vi "MC collect shot data from tcp queue.vi"(6 "Scan.ShotDataQueuesAndEvents.tcp data event":T1, 7 "TCP subscriptions info":T2, 8 "error in (no error)":errorcluster, 9 "timeout for get all devs (ms)":u32=5000, 10 "ScanData event reg ref":refnum<event-registration>, 11 "TCPshotDataQueue":refnum<queue>) -> (0 "error out":errorcluster, 1 "timeout":bool, 2 "device times":cluster{"Device":string, "time":u32}[](array[cluster]), 3 "All data out":string[][](array[string]))   [LabVIEW 2020]
uses:
  Shared/GUI_Template/TCP subscription info cluster.ctl
  Shared/GUI_Template/GUI_master/tcp_new_data_event.ctl
  Shared/GUI_Template/GUI_master/tcp new data cluster.ctl
panel:
  out "number of events discarded":u32
  out "device times all data received":cluster{"Device":string, "time":u32}[](array[cluster])
  out "dev times timeout":cluster{"Device":string, "time":u32}[](array[cluster])
  out "time waited":u32(graph)
  out "timeout":bool
  out "time":u32 caption="time waiting"
  out "Devs no data":string[](array[string])
  out "loop time":u32
  out "Device name":string
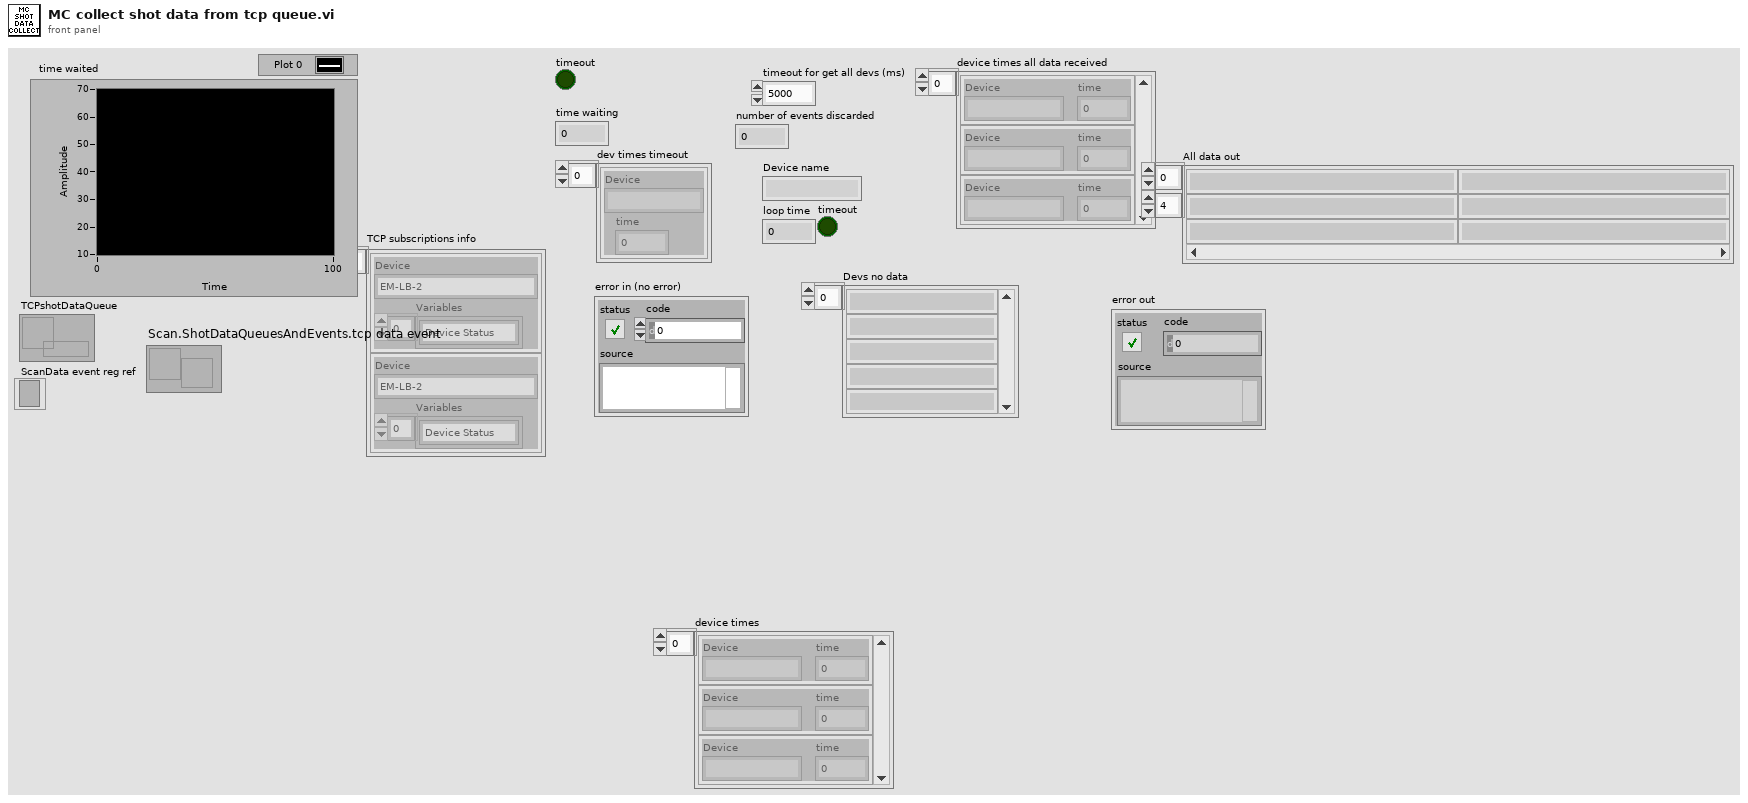
[diagram p1: front panel]
types:
  T1 = typedef "tcp_new_data_event.ctl" = refnum<user-event>
  T2 = typedef "TCP subscription info cluster.ctl" = cluster{"Device":string, "Variables":string[]}[]
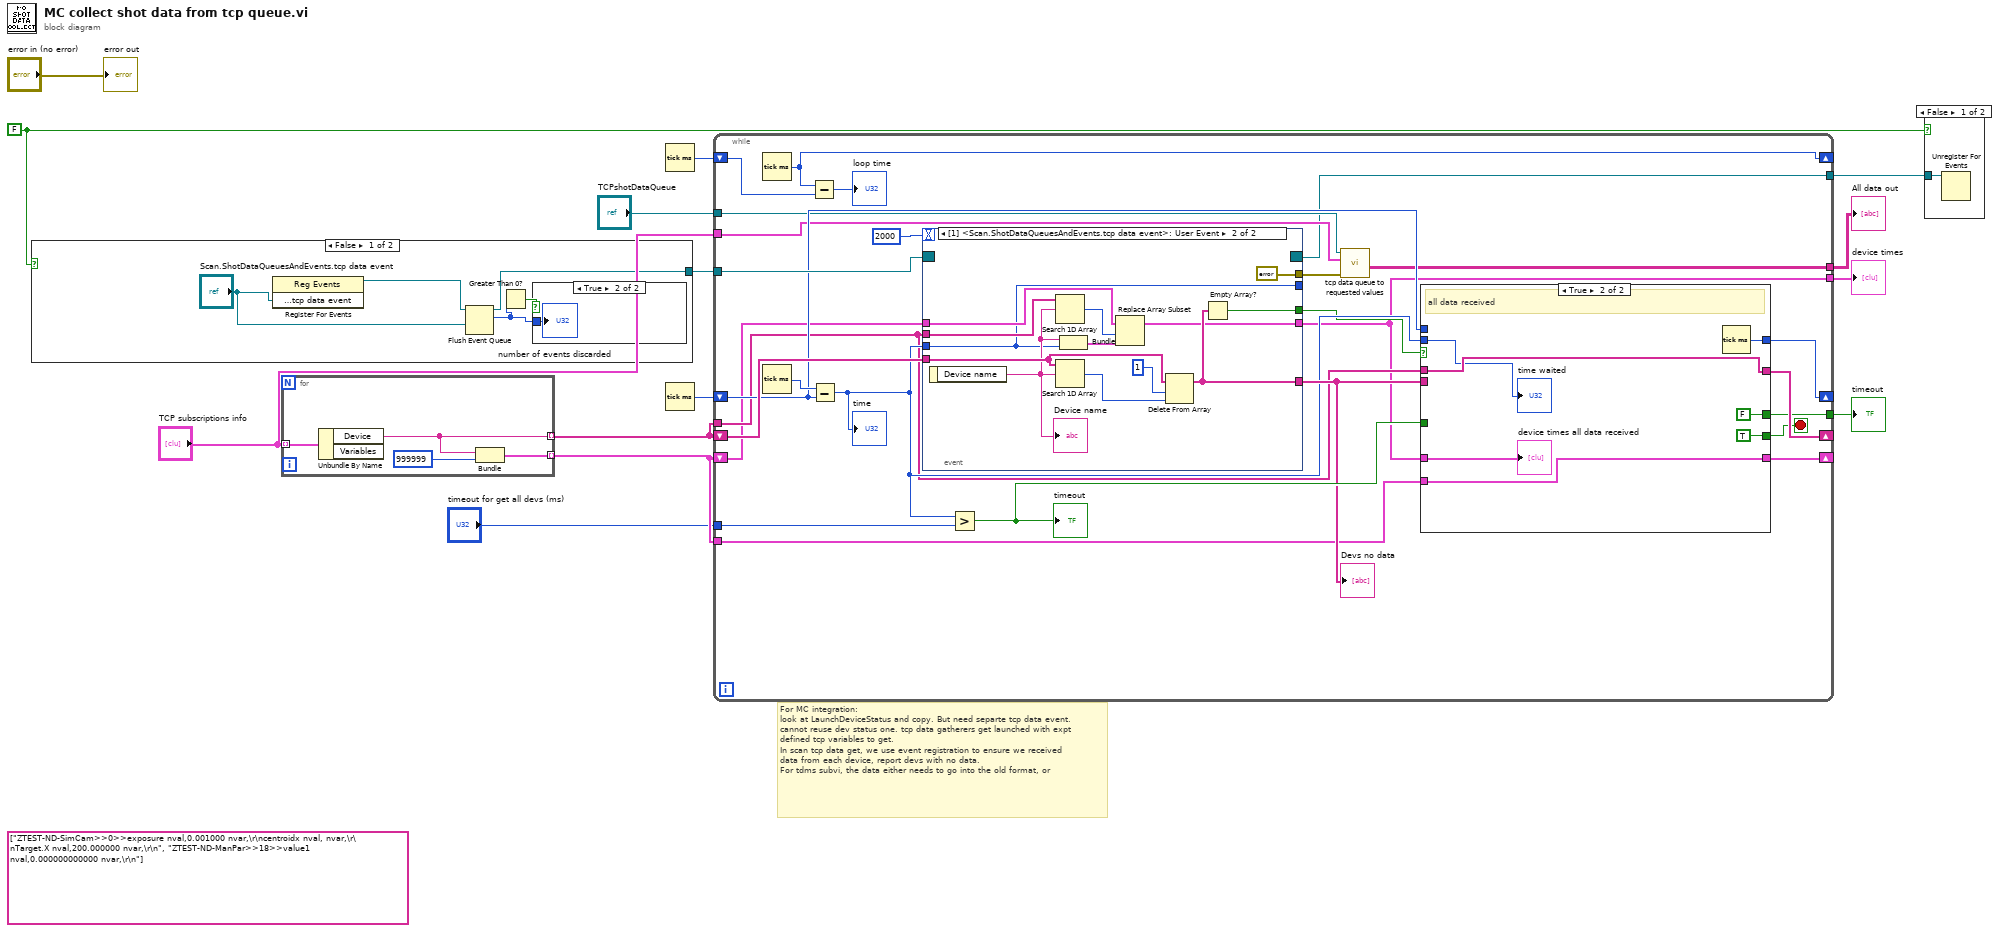
[diagram p0: block diagram]
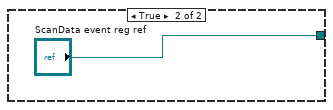
[diagram p3: hidden frame]
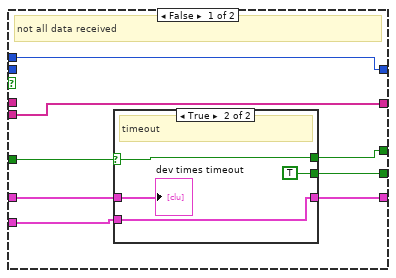
[diagram p5: hidden frame]
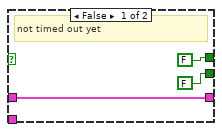
[diagram p6: hidden frame]
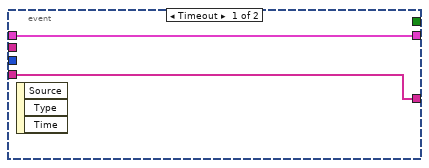
[diagram p7: hidden frame]
diagram:
  w2 = FALSE
  (unwired) string[] ["ZTEST-ND-SimCam>>0>>exposure nval,0.001000 nvar,\r\ncentroidx nval, nvar,\r\nTarget.X nval,200.000000 nvar,\r\n", "ZTEST-ND-ManPar>>18>>value1 nval,0.000000000000 nvar,\r\n"] ("Scan data in")
  # "For MC integration:\nlook at LaunchDeviceStatus and copy. But need separte tcp data event. cannot reuse dev status one. tcp data gatherers get launched with expt defined tcp variables to get.\nIn scan tcp data get, we use event registration to ensure we received data from each device, report devs with no data.\nFor tdms subvi, the data either needs to go into the old format, or"
  n1 = case shown="False" w2 {
    tunnel: [w17 "ScanData event reg ref"] -> w3
    frame False {
      n2 = register-events("Scan.ShotDataQueuesAndEvents.tcp data event") -> (reference out=w19:refnum<event-registration>)  [unwired: 2 in, 1 out]
      n3 = Flush Event Queue(0:w19, 2:"Scan.ShotDataQueuesAndEvents.tcp data event") -> (8:w17:refnum<event-registration>, 9:w16:u32)  [unwired: 4 in, 1 out]
      n4 = Greater Than 0?(x=w16) -> (x > 0?=w15:bool)
      n5 = case shown="True" w15 {
        tunnel: w16 -> [_ w20]
        frame False {
        }
        frame True {
          "number of events discarded" <- w20
        }
      }
    }
    frame True {
    }
  }
  n6 = for {
    tunnel: "TCP subscriptions info" -> [w25] mode=indexing
    tunnel: [w24] -> w12 mode=indexing
    tunnel: [w22] -> w10 mode=indexing
    n7 = Unbundle By Name(w25) -> ("Device"=w24:string)  [unwired: 1 out]
    n8 = Bundle("Device"=w24, "time"=u32 999999) -> (w22:cluster{"Device":string, "time":u32})  [unwired: 1 in]
  }
  n9 = Tick Count (ms)() -> (millisecond timer value=w14:u32)
  n10 = Tick Count (ms)() -> (millisecond timer value=w11:u32)
  n11 = while {
    tunnel: "TCPshotDataQueue" -> [w31]
    tunnel: "TCP subscriptions info" -> [w32]
    tunnel: w3 -> [w52]
    shift-right: [w50] -> _
    shift-left: w14 -> [w49]
    shift-right: [w41] -> _
    shift-left: w12 -> [w47]
    tunnel: w12 -> [w39]
    shift-right: [w45] -> _
    shift-left: w11 -> [w44]
    shift-right: [w36] -> _
    shift-left: w10 -> [w38]
    tunnel: w10 -> [w37]
    tunnel: "timeout for get all devs (ms)" -> [w34]
    tunnel: [w30] -> w4
    tunnel: [w29] -> w7
    tunnel: [w28] -> w5
    tunnel: [w27] -> w1
    stop <- w33 stop-if-true
    n12 = Tick Count (ms)() -> (millisecond timer value=w50:u32)
    n13 = Tick Count (ms)() -> (millisecond timer value=w46:u32)
    n14 = Subtract(x=w50, y=w49) -> (x-y=→"loop time":u32)
    n15 = Subtract(x=w46, y=w44) -> (x-y=w40:u32)
    "time" <- w40
    n16 = event shown="[1] <Scan.ShotDataQueuesAndEvents.tcp data event>: User Event" {
      selector: w52 -> [_ _]
      dyn-events: [_ _] -> w27
      timeout: 2000 -> [_ _]
      tunnel: w47 -> [w76 w87]
      tunnel: [w76 w86] -> w42
      tunnel: [_ w85] -> w35
      tunnel: [_ w80] -> _
      tunnel: w40 -> [_ w80]
      tunnel: w39 -> [_ w84]
      tunnel: w38 -> [w75 w83]
      tunnel: [w75 w78] -> w29
      tunnel: [_ errorcluster {"status"=FALSE, "code"=0, "source"=""} ("error in (no error)")] -> w26
      event Timeout {
        n17 = event-data() -> ()  [unwired: 1 in, 3 out]
      }
      event User Event {
        n18 = event-data() -> ("Device name"=w82:string)  [unwired: 1 in]
        "Device name" <- w82
        n19 = Search 1D Array(1D array=w84, element=w82) -> (index of element=w81:i32)  [unwired: 1 in]
        n20 = Search 1D Array(1D array=w87, element=w82) -> (index of element=w89:i32)  [unwired: 1 in]
        n21 = Bundle("Device name"=w82, w80) -> (w79:cluster{"Device name":string, u32})  [unwired: 1 in]
        n22 = Replace Array Subset(array=w83, new element=w79, index=w81) -> (w78:cluster{"Device":string, "time":u32}[])
        n23 = Delete From Array(array=w87, length=1, index=w89) -> (array with subset deleted=w86:string[])  [unwired: 1 out]
        n24 = Empty Array?(array=w86) -> (empty?=w85:bool)
      }
    }
    "Devs no data" <- w42
    n25 = Greater?(x=w40, y=w34) -> (0:w43:bool)
    "timeout" <- w43
    n26 = call "tcp data queue to requested values.vi"("error in (no error)"=w26, "TCP subscriptions info"=w32, "Queue in"=w31) -> ("All data"=w30:string[][])  [unwired: 5 in, 3 out]
    n27 = case shown="True" w35 {
      tunnel: [w60 w74] -> w45
      tunnel: w44 -> [w60 _]
      tunnel: w43 -> [w59 _]
      tunnel: w39 -> [_ w73]
      tunnel: w42 -> [w58 _]
      tunnel: [w58 w73] -> w41
      tunnel: w40 -> [_ w72]
      tunnel: w29 -> [w57 w71]
      tunnel: w37 -> [w55 w70]
      tunnel: [w56 w70] -> w36
      tunnel: [w54 TRUE] -> w33
      tunnel: [w53 FALSE] -> w28
      frame False {
        # "not all data received"
        n28 = case shown="True" w59 {
          selector: w59 -> [_ w64]
          tunnel: w57 -> [w63 w67]
          tunnel: [w63 w66] -> w56
          tunnel: w55 -> [_ w66]
          tunnel: [FALSE TRUE] -> w54
          tunnel: [FALSE w64] -> w53
          frame False {
            # "not timed out yet"
          }
          frame True {
            # "timeout"
            "dev times timeout" <- w67
          }
        }
      }
      frame True {
        # "all data received"
        n29 = Tick Count (ms)() -> (millisecond timer value=w74:u32)
        "time waited" <- w72
        "device times all data received" <- w71
      }
    }
  }
  "All data out" <- w4
  "device times" <- w7
  "timeout" <- w5
  n30 = case shown="False" w2 {
    tunnel: w1 -> [w90 _]
    frame False {
      n31 = Unregister For Events(event registration refnum=w90) -> ()  [unwired: 1 in, 1 out]
    }
    frame True {
    }
  }
  "error out" <- "error in (no error)"
